vi "VI Tree.vi"   [LabVIEW 2011, in "DMM4.lvlib"]
doc: "This is the instrument driver for the <INSTRUMENT NAME>. The VI Tree displays all the user-callable VIs of the instrument driver in an organized table."
uses:
  <instrlib>/DMM4/DMM4.lvlib
panel:
  # "SEE DIAGRAM\nFOR VI TREE."
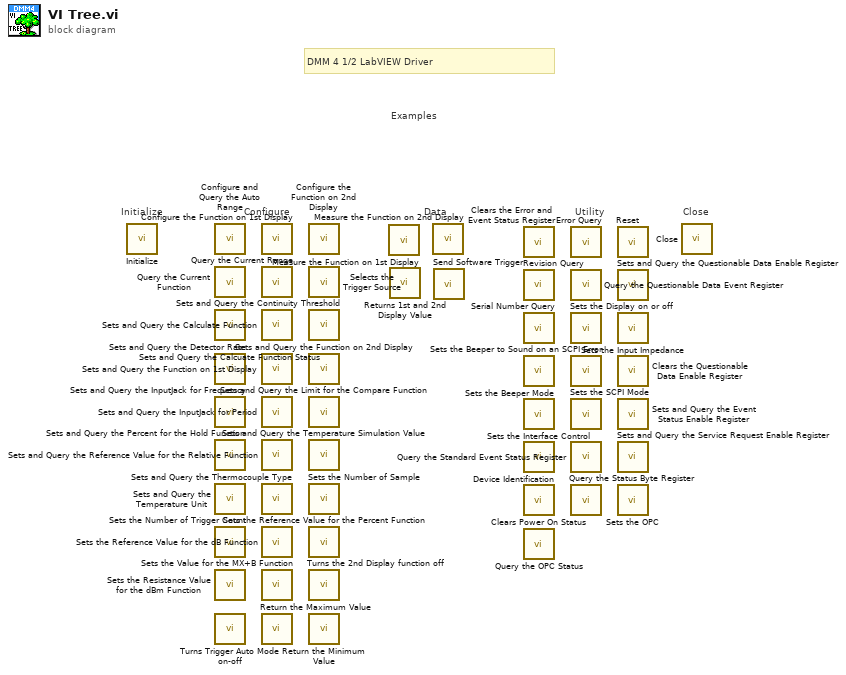
[diagram p0: block diagram]
diagram:
  # "Examples"
  # "DMM 4 1/2 LabVIEW Driver"
  # "Configure"
  # "Utility"
  # "Data"
  # "Close"
  # "Initialize"
  n1 = call <instrlib>:"Initialize.vi"() -> ()  [unwired: 8 in, 4 out]
  n2 = call <instrlib>:"Configure and Query the Auto Range.vi"() -> ()  [unwired: 9 in, 3 out]
  n3 = call <instrlib>:"Query the Current Function.vi"() -> ()  [unwired: 9 in, 3 out]
  n4 = call <instrlib>:"Sets and Query the Calcuate Function Status.vi"() -> ()  [unwired: 9 in, 3 out]
  n5 = call <instrlib>:"Sets and Query the Detector Rate.vi"() -> ()  [unwired: 9 in, 3 out]
  n6 = call <instrlib>:"Sets and Query the InputJack for Frequency.vi"() -> ()  [unwired: 9 in, 3 out]
  n7 = call <instrlib>:"Sets and Query the Percent for the Hold Function.vi"() -> ()  [unwired: 9 in, 3 out]
  n8 = call <instrlib>:"Sets and Query the Temperature Unit.vi"() -> ()  [unwired: 9 in, 3 out]
  n9 = call <instrlib>:"Sets the Number of Trigger Count.vi"() -> ()  [unwired: 9 in, 3 out]
  n10 = call <instrlib>:"Sets the Resistance Value for the dBm Function.vi"() -> ()  [unwired: 9 in, 3 out]
  n11 = call <instrlib>:"Turns Trigger Auto Mode on-off.vi"() -> ()  [unwired: 9 in, 3 out]
  n12 = call <instrlib>:"Configure the Function on 1st Display .vi"() -> ()  [unwired: 10 in, 2 out]
  n13 = call <instrlib>:"Query the Current Range.vi"() -> ()  [unwired: 9 in, 3 out]
  n14 = call <instrlib>:"Sets and Query the Calculate Function.vi"() -> ()  [unwired: 10 in, 2 out]
  n15 = call <instrlib>:"Sets and Query the Function on 1st Display.vi"() -> ()  [unwired: 9 in, 3 out]
  n16 = call <instrlib>:"Sets and Query the InputJack for Period.vi"() -> ()  [unwired: 9 in, 3 out]
  n17 = call <instrlib>:"Sets and Query the Reference Value for the Relative Function.vi"() -> ()  [unwired: 9 in, 3 out]
  n18 = call <instrlib>:"Sets and Query the Thermocouple Type.vi"() -> ()  [unwired: 9 in, 3 out]
  n19 = call <instrlib>:"Sets the Reference Value for the dB Function.vi"() -> ()  [unwired: 9 in, 3 out]
  n20 = call <instrlib>:"Sets the Value for the MX+B Function.vi"() -> ()  [unwired: 8 in, 4 out]
  n21 = call <instrlib>:"Return the Maximum Value.vi"() -> ()  [unwired: 9 in, 3 out]
  n22 = call <instrlib>:"Configure the Function on 2nd Display.vi"() -> ()  [unwired: 10 in, 2 out]
  n23 = call <instrlib>:"Selects the Trigger Source.vi"() -> ()  [unwired: 9 in, 3 out]
  n24 = call <instrlib>:"Sets and Query the Continuity Threshold.vi"() -> ()  [unwired: 10 in, 2 out]
  n25 = call <instrlib>:"Sets and Query the Function on 2nd Display.vi"() -> ()  [unwired: 9 in, 3 out]
  n26 = call <instrlib>:"Sets and Query the Limit for the Compare Function.vi"() -> ()  [unwired: 8 in, 4 out]
  n27 = call <instrlib>:"Sets and Query the Temperature Simulation Value.vi"() -> ()  [unwired: 9 in, 3 out]
  n28 = call <instrlib>:"Sets the Number of Sample.vi"() -> ()  [unwired: 9 in, 3 out]
  n29 = call <instrlib>:"Sets the Reference Value for the Percent Function.vi"() -> ()  [unwired: 9 in, 3 out]
  n30 = call <instrlib>:"Turns the 2nd Display function off.vi"() -> ()  [unwired: 10 in, 2 out]
  n31 = call <instrlib>:"Return the Minimum Value.vi"() -> ()  [unwired: 9 in, 3 out]
  n32 = call <instrlib>:"Measure the Function on 1st Display.vi"() -> ()  [unwired: 9 in, 3 out]
  n33 = call <instrlib>:"Returns 1st and 2nd Display Value.vi"() -> ()  [unwired: 9 in, 3 out]
  n34 = call <instrlib>:"Measure the Function on 2nd Display.vi"() -> ()  [unwired: 9 in, 3 out]
  n35 = call <instrlib>:"Send Software Trigger.vi"() -> ()  [unwired: 10 in, 2 out]
  n36 = call <instrlib>:"Clears the Error and Event Status Register.vi"() -> ()  [unwired: 10 in, 2 out]
  n37 = call <instrlib>:"Revision Query.vi"() -> ()  [unwired: 8 in, 4 out]
  n38 = call <instrlib>:"Serial Number Query.vi"() -> ()  [unwired: 9 in, 3 out]
  n39 = call <instrlib>:"Sets the Beeper Mode.vi"() -> ()  [unwired: 9 in, 3 out]
  n40 = call <instrlib>:"Sets the Interface Control.vi"() -> ()  [unwired: 10 in, 2 out]
  n41 = call <instrlib>:"Device Identification.vi"() -> ()  [unwired: 9 in, 3 out]
  n42 = call <instrlib>:"Clears Power On Status.vi"() -> ()  [unwired: 12 in]
  n43 = call <instrlib>:"Query the OPC Status.vi"() -> ()  [unwired: 9 in, 3 out]
  n44 = call <instrlib>:"Error Query.vi"() -> ()  [unwired: 9 in, 3 out]
  n45 = call <instrlib>:"Query the Questionable Data Event Register.vi"() -> ()  [unwired: 9 in, 3 out]
  n46 = call <instrlib>:"Sets the Display on or off.vi"() -> ()  [unwired: 9 in, 3 out]
  n47 = call <instrlib>:"Sets the Beeper to Sound on an SCPI Error.vi"() -> ()  [unwired: 9 in, 3 out]
  n48 = call <instrlib>:"Sets the SCPI Mode.vi"() -> ()  [unwired: 10 in, 2 out]
  n49 = call <instrlib>:"Query the Standard Event Status Register.vi"() -> ()  [unwired: 9 in, 3 out]
  n50 = call <instrlib>:"Query the Status Byte Register.vi"() -> ()  [unwired: 10 in, 2 out]
  n51 = call <instrlib>:"Reset.vi"() -> ()  [unwired: 10 in, 2 out]
  n52 = call <instrlib>:"Sets and Query the Questionable Data Enable Register.vi"() -> ()  [unwired: 9 in, 3 out]
  n53 = call <instrlib>:"Sets the Input Impedance.vi"() -> ()  [unwired: 9 in, 3 out]
  n54 = call <instrlib>:"Clears the Questionable Data Enable Register.vi"() -> ()  [unwired: 10 in, 2 out]
  n55 = call <instrlib>:"Sets and Query the Event Status Enable Register.vi"() -> ()  [unwired: 9 in, 3 out]
  n56 = call <instrlib>:"Sets and Query the Service Request Enable Register.vi"() -> ()  [unwired: 9 in, 3 out]
  n57 = call <instrlib>:"Sets the OPC.vi"() -> ()  [unwired: 10 in, 2 out]
  n58 = call <instrlib>:"Close.vi"() -> ()  [unwired: 11 in, 1 out]
